vi "Mouse Move.vi"(8 "error in (no error)":errorcluster, 11 "ScrollingList in":refnum<class "ScrollingList.lvclass">) -> (0 "error out":errorcluster, 3 "ScrollingList (dup)":refnum<class "ScrollingList.lvclass">)   [LabVIEW 2020, in "ScrollingList.lvclass"]
uses:
  ScrollingList.lvclass
  C:/Program Files/National Instruments/LabVIEW 2020/vi.lib/QSI/QControls/QControl Classes/Picture/Picture.lvclass
  ScrollingList.lvclass/ScrollingList.ctl
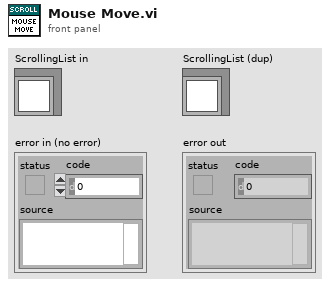
[diagram p1: front panel]
types:
  T1 = typedef "ScrollingList.lvclass/State Data.ctl" = cluster{"Timeout":i32, "Time":timestamp, "Y":i32, "Origin:Top":i16, "Rate":dbl, "ListItems":string[], "Item Height":i32, "Max Height":i32}
  T2 = typedef "LVMouseTypeDef.ctl" = cluster{"Mouse Position":cluster{"X":i32, "Y":i32}, "Mouse Modifiers":cluster{"Button Down":bool, "Shift Mod":bool, "Menu Mod":bool, "Option Mod":bool}}
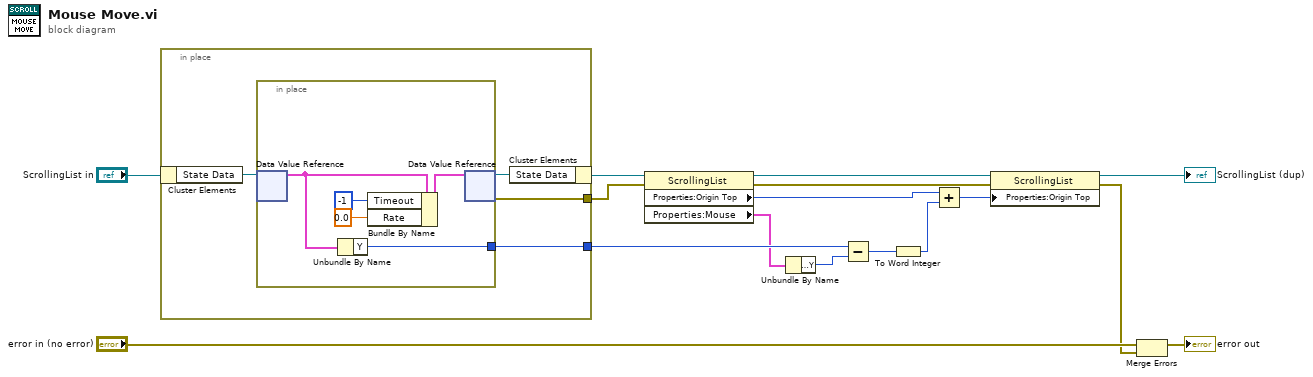
[diagram p0: block diagram]
diagram:
  n1 = in-place {
    in-place-border: [w18] -> w12
    in-place-border: [w17] -> w5
    n2 = in-place-cluster #1("ScrollingList in") -> ("State Data"=w20:refnum<data-value>)
    n3 = in-place {
      in-place-border: [w21] -> w18
      n4 = in-place-dvr #2(w20) -> (w22:T1)  [unwired: 1 out]
      n5 = Unbundle By Name(w22) -> ("Y"=w21:i32)
      n6 = Bundle By Name(cluster=w22, "Timeout"=-1, "Rate"=0.0) -> (w25:T1)
      n7 = in-place-dvr #2(w25) -> (w19:refnum<data-value>, w17:errorcluster)
    }
    n8 = in-place-cluster #1("State Data"=w19) -> (w15:refnum<class "ScrollingList.lvclass">)
  }
  n9 = property on="Property Node" class="ScrollingList"(reference=w15, error in=w5) -> (reference out=w14:refnum<class "ScrollingList.lvclass">, error out=w4:errorcluster, "Properties:Origin Top"=w8:i16, "Properties:Mouse"=w6:T2)
  n10 = Unbundle By Name(w6) -> ("Mouse Position.Y"=w11:i32)
  n11 = Subtract(x=w12, y=w11) -> (x-y=w10:i32)
  n12 = To Word Integer(number=w10) -> (16bit integer=w9:i16)
  n13 = Add(x=w8, y=w9) -> (x+y=w7:i16)
  n14 = property on="Property Node" class="ScrollingList"(reference=w14, error in=w4, "Properties:Origin Top"=w7) -> (reference out=→"ScrollingList (dup)":refnum<class "ScrollingList.lvclass">, error out=w1:errorcluster)
  n15 = Merge Errors("error in (no error)", w1) -> (→"error out":errorcluster)
